vi "data_IO_tinius.vi"() -> ()   [LabVIEW 2023]
uses:
  <vilib>/DAQmx/read.llb/DAQmx Read (Analog DBL 1Chan 1Samp).vi
  <vilib>/DAQmx/create/channels.llb/DAQmx Create Channel (AI-Voltage-Basic).vi
  <vilib>/DAQmx/configure/timing.llb/DAQmx Timing (Sample Clock).vi
  <vilib>/DAQmx/miscellaneous.llb/DAQmx Fill In Error Info.vi
panel:
  out "Force":dbl(graph)
  in  "stop":bool
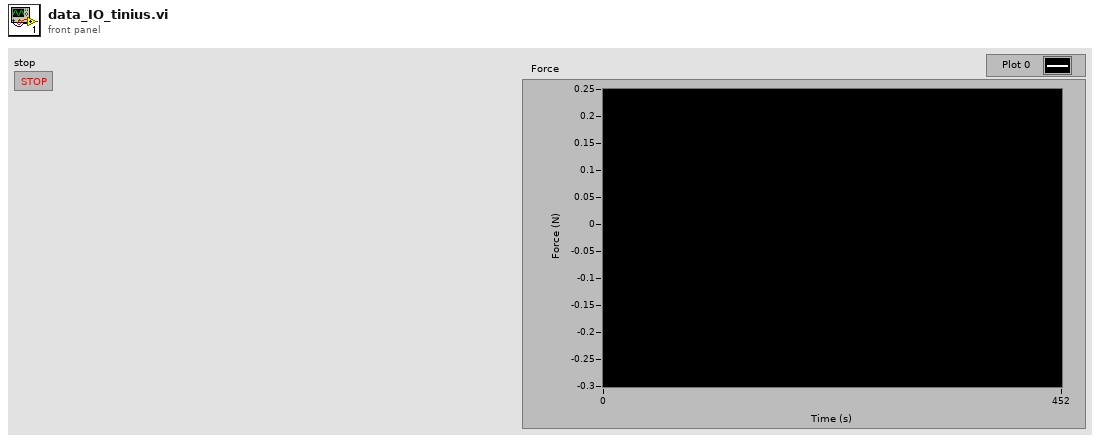
[diagram p1: front panel]
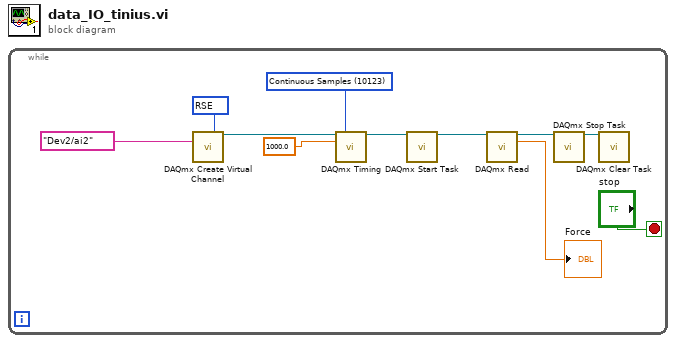
[diagram p0: block diagram]
diagram:
  n1 = while {
    stop <- "stop" stop-if-true
    w8 = 10123 items=["Finite Samples"=10178, "Continuous Samples"=10123, "Hardware Timed Single Point"=12522] ("sample mode")
    w6 = 10083 items=["Default"=-1, "RSE"=10083, "NRSE"=10078, "Differential"=10106, "Pseudodifferential"=12529] ("input terminal configuration")
    n2 = call-poly <vilib>:"DAQmx Create Virtual Channel.vi"("input terminal configuration"=w6, "physical channels"=tag "Dev2/ai2") -> ("task out"=w9:refnum<k21>)  [unwired: 12 in, 1 out]
    n3 = call-poly <vilib>:"DAQmx Timing.vi"("task/channels in"=w9, "sample mode"=w8, "rate"=1000.0) -> ("task out"=w1:refnum<k21>)  [unwired: 11 in, 1 out]
    n4 = call <vilib>:"DAQmx Start Task.vi"("task/channels in"=w1) -> ("task out"=w2:refnum<k21>)  [unwired: 13 in, 1 out]
    n5 = call-poly <vilib>:"DAQmx Read.vi"("task/channels in"=w2) -> ("task out"=w4:refnum<k21>, "data"=→"Force":dbl)  [unwired: 12 in, 1 out]
    n6 = call <vilib>:"DAQmx Stop Task.vi"("task/channels in"=w4) -> ("task out"=w3:refnum<k21>)  [unwired: 13 in, 1 out]
    n7 = call <vilib>:"DAQmx Clear Task.vi"("task in"=w3) -> ()  [unwired: 14 in, 1 out]
  }
